vi "cw_2_1.vi"() -> ()   [LabVIEW 2022 SP3]
uses:
  <vilib>/numeric/Random Number (Range) I64.vi
  <vilib>/numeric/sub_Random U32.vi
panel:
  in  "noise amplitude":dbl=30.0
  in  "frequency":dbl=2.0
  out "time":dbl
  out "Waveform Chart":dbl(graph)
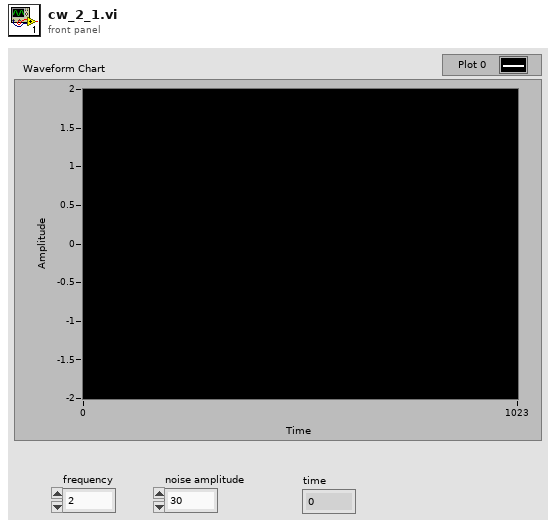
[diagram p1: front panel]
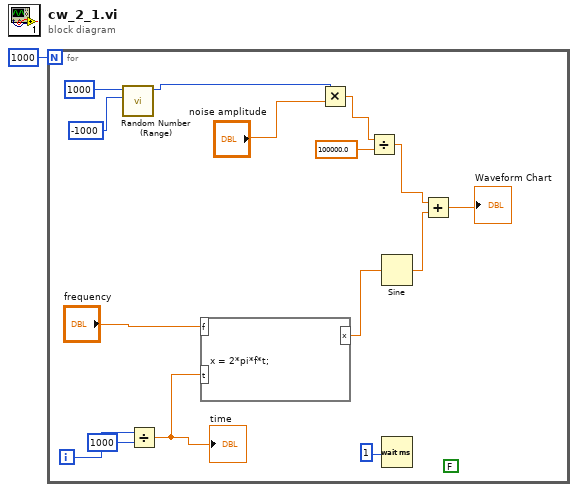
[diagram p0: block diagram]
diagram:
  n1 = for {
    N: 1000 -> [_]
    i -> [w16]
    (unwired) FALSE
    n2 = call-poly <vilib>:"Random Number (Range).vi"("lower bound (-100)"=i64 -1000, "upper bound (100)"=i64 1000) -> ("number"=w5:i64)  [unwired: 9 in]
    n3 = Divide(x=w16, y=1000) -> (x/y=w13:dbl)
    "time" <- w13
    n4 = formula code="x = 2*pi*f*t;"("f"="frequency", "t"=w13) -> ("x"=w14:dbl)
    n5 = Multiply(x=w5, y="noise amplitude") -> (x*y=w4:dbl)
    n6 = Divide(x=w4, y=100000.0) -> (x/y=w3:dbl)
    n7 = Sine(x=w14) -> (sin(x)=w8:dbl)
    n8 = Wait (ms)(milliseconds to wait=u32 1) -> ()  [unwired: 1 out]
    n9 = Add(x=w3, y=w8) -> (x+y=→"Waveform Chart":dbl)
  }
